vi "SSH.vi"(10 "Udkast array":i32[](array[numeric]), 11 "Andtal kast":i32) -> (3 "Probabilitets array":dbl[](array[numeric]))   [LabVIEW 2022 SP3]
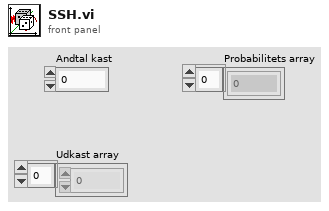
[diagram p1: front panel]
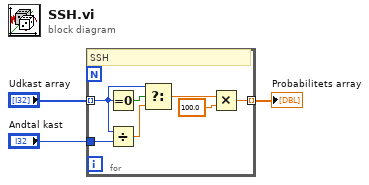
[diagram p0: block diagram]
diagram:
  n1 = for {
    tunnel: "Udkast array" -> [w7] mode=indexing
    tunnel: "Andtal kast" -> [w8]
    tunnel: [w4] -> w3 mode=indexing
    # "SSH"
    n2 = Equal To 0?(x=w7) -> (x = 0?=w10:bool)
    n3 = Divide(x=w7, y=w8) -> (x/y=w9:dbl)
    n4 = Select(t=w7, s=w10, f=w9) -> (s? t:f=w5:dbl)
    n5 = Multiply(x=w5, y=100.0) -> (x*y=w4:dbl)
  }
  "Probabilitets array" <- w3
